vi "play-raster-scan-with-SOS-ID.vi"() -> ()   [LabVIEW 2017]
uses:
  raster-scan-params.ctl
  controls/PI-params.ctl
  controls/boolean_info.ctl
  controls/raster_input_meta_data.ctl
  <vilib>/userdefined/High Color/nirio_resource_hc.ctl
  controls/rasterMetaData.ctl
  <vilib>/Utility/file.llb/Read Delimited Spreadsheet (DBL).vi
  <vilib>/FPGAPlugInAG/cRIO-9082/niLvFpga_Open_cRIO-9082.vi
  <vilib>/rvi/interface/common/dynamic/niFpgaDynamicAddResources.vi
  <vilib>/FPGAPlugInAG/Dynamic/niLvFpga_Reset_Dynamic.vi
  <vilib>/rvi/interface/common/niFpgaWaitOnOcc.vi
  <vilib>/Utility/error.llb/Error Cluster From Error Code.vi
  <vilib>/rvi/errors/niLvFpgaAdjustHostInterfaceError.vi
  <vilib>/FPGAPlugInAG/Dynamic/niLvFpga_Run_Dynamic.vi
  fpga_interface_lib/acquire_FXP_16-5_FIFO_2.vi
  <vilib>/FPGAPlugInAG/Dynamic/niLvFpga_Close_Dynamic.vi
  <userlib>/_matio/level5/Public/Write/Append Data Element.llb/Append Data Element (Anything).vi
  <vilib>/rvi/interface/nirviOpenFPGA/nirviOpenFPGA.xnode
  FPGA Bitfiles/afmimagingcontro_FPGATargetSPARTA_raster-scanning_ejZpyk2O7fU.lvbitx
  <vilib>/rvi/interface/nirviMethod/nirviMethod.xnode
  <vilib>/rvi/interface/nirviReadWriteControl/nirviReadWriteControl.xnode
  <vilib>/rvi/interface/nirviCloseFPGA/nirviCloseFPGA.xnode
  <vilib>/FPGAPlugInAG/Dynamic/niLvFpga_ConfigureFifo_Dynamic.vi
  <vilib>/rvi/errors/niLvFpgaMergeErrorWithErrorCode.vi
  <vilib>/rvi/interface/Simulation/niFpgaSimulationCallBeginRW.vi
  fpga_interface_lib/fpga_interface.lvlib
  NiFpgaLv.dll
  <userlib>/_matio/level5.lvlib
  <vilib>/FPGAPlugInAG/Dynamic/niLvFpga_WriteFifo_Dynamic.vi
panel:
  in  "Ring 2":u16(ring) items=["x(k)", "y(k)", "deflection", "u_z"]
  in  "Alert-on-Finish":bool
  in  "do-Dz":bool
  in  "KI_derate":sgl
  in  "ze_sched_thresh":sgl
  in  "detrend":bool=TRUE
  out "InputMetaData":T1
  out "output-meta-data-path":path
  out "Tab Control":T2(tab)
  in  "Amplitude":dbl=0.15 format="%#_13g"
  in  "Swept-Sines-Control-Settings":cluster{"u-max":sgl, "offset":sgl, "Ki":sgl}
  out "Bode amplitude":cluster{"W":dbl[], "Magnitude":dbl[]}[](graph) caption="Magnitude Graph"
  in  "input-path":path=path "Z:/afm-cs/imaging/raster/5microns/parents/raster_scan_512pix_5mic_01Hz.csv"
  in  "number-of-pixels":i32=512
  out "points_per_line":i32=250000
  out "total_num_points":i32
  in  "raise-constant (init)":sgl
  in  "raise-constant":sgl
  in  "trigger-0":bool
  in  "STOP":bool
  in  "xy-init":fxp<+/-,16,5>[](array[numeric])=[0.0, 0.0]
  in  "Ki-xy":dbl=0.015 format="%#_13g"
  out "ADC-zaxis":sgl
  out "DAC-zaxis":sgl
  in  "xy-bound":sgl=7.0
  out "output-data-path":path
  in  "note-blob":string
  in  "overwrite":bool
  in  "raster-scan-params":T3={"TsTicks"=1600, "Stop"=FALSE, "TOL"=0.3, "ramp-rate"=-0.0002, "z-u-max"=5.0, "PI-params"={"Ki"=0.01, "setpoint"=-0.3}, "Num"=[1.0237086, -2.0434425, 1.0225973, 0.0, 0.0, 0.0, 0.0, 0.0, 0.0], "TF Order"=2, "Den"=[1.0, -1.9961116, 0.998975, 0.0, 0.0, 0.0, 0.0, 0.0, 0.0]} {"ramp-rate" format="%#_5g"; "TOL" format="%#_13g"}
  in  "do_xy_CL":bool=TRUE
  out "boolean errors":T5
  in  "Z-settle-N":i16=10000
  out "Actual Depth":u32
  out "Elements Remaining":u32
  out "size(s)":i32
  out "y iter":i32
  out "nsamps 2":i32
  out "Empty Elements Remaining":u32
  out "(int) y*floor(x/y)":u64
  out "elements left 2":i32=1
  out "x >= y?":bool
  out "writing stopped":bool
  out "size(s) 2":i32
  out "case-selector-feedback":i16
  out "e(0) (threshhold init)":fxp<+/-,16,5>
  out "que timed out?":bool
  out "base y_ref (ramp)":dbl[](graph)
  out "base x_ref(triangle wave)":dbl[](graph)
  out "error":dbl[](graph)
  out "control":dbl[](graph)
  out "x":dbl[](graph)
  out "total-time":dbl
  out "Error signal (previous line) 2":dbl[](graph)
  out "Waveform Graph":dbl[](graph)
  out "Intensity Graph":dbl[][](graph)
  out "control signal (previous line)":dbl[](graph)
  # "x-axis"
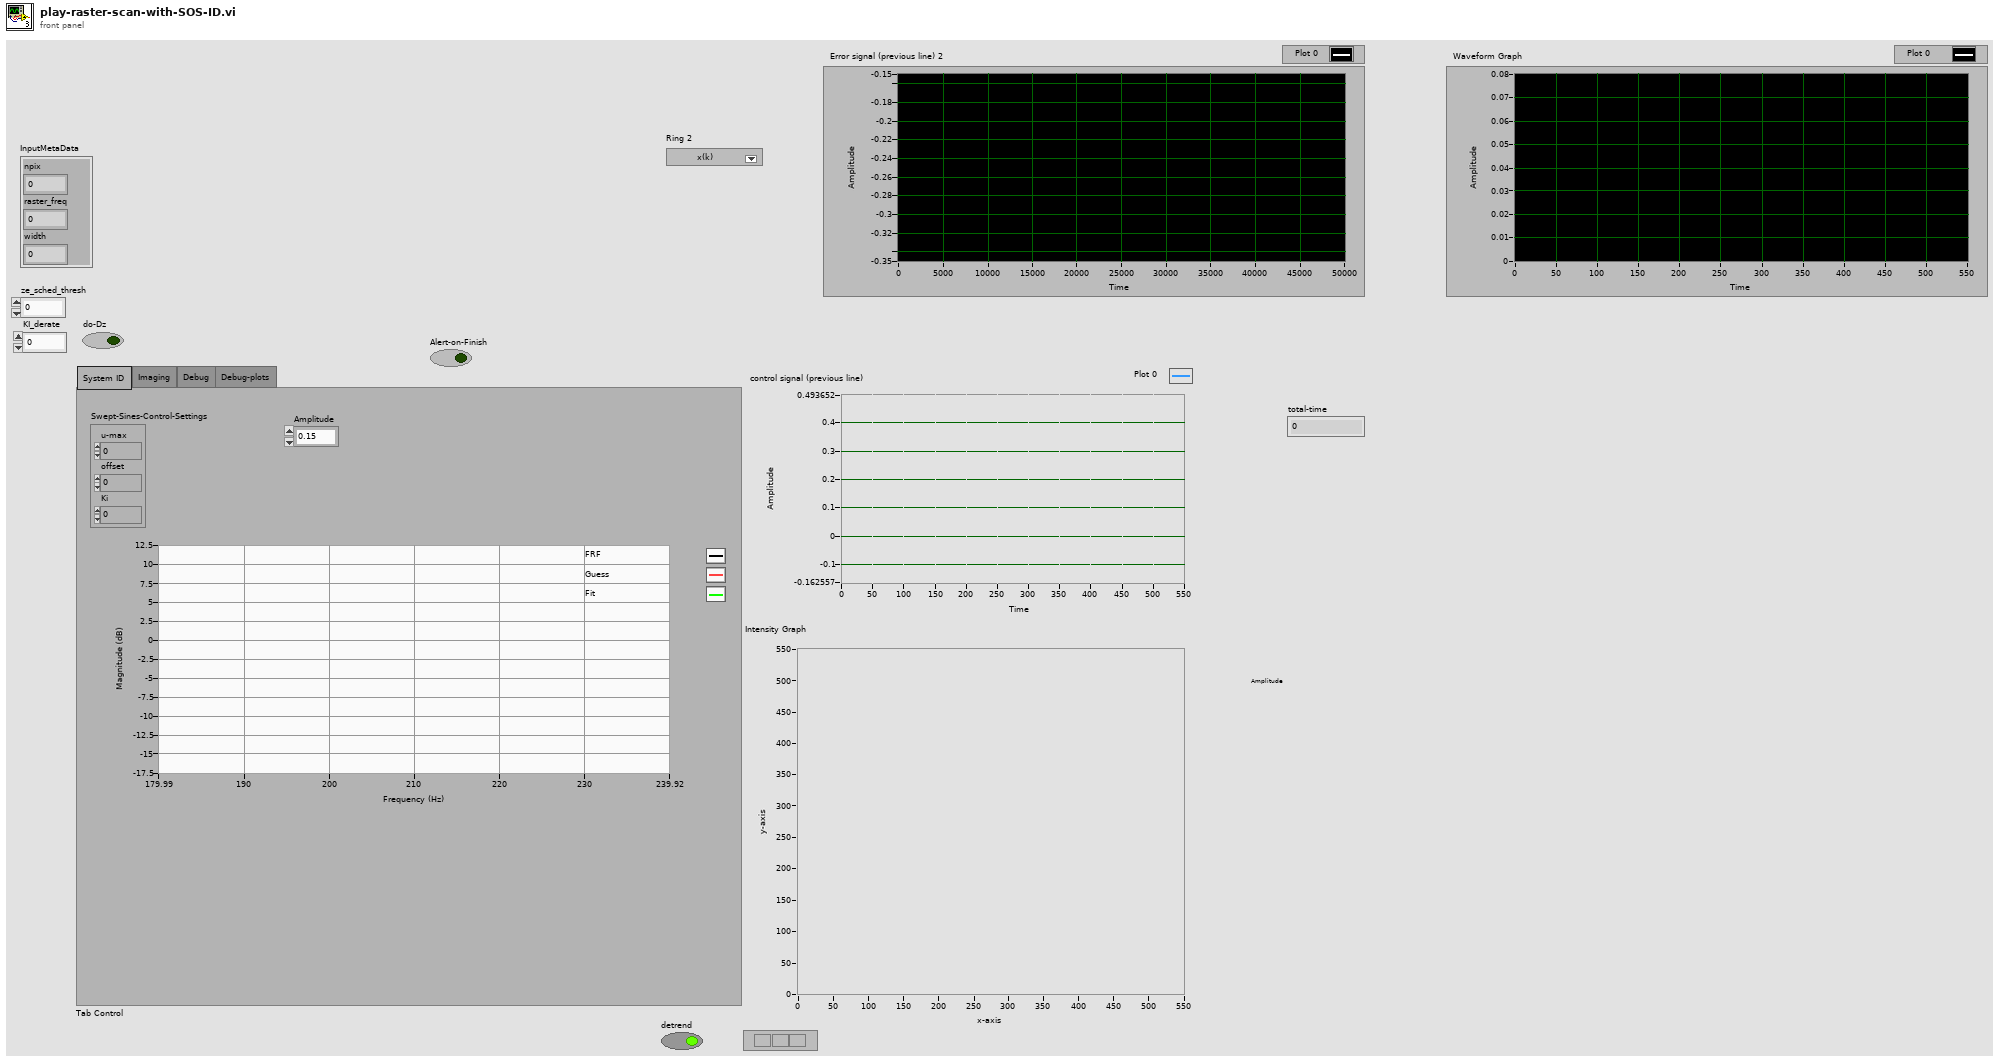
[diagram p1: front panel]
types:
  T1 = typedef "raster_input_meta_data.ctl" = cluster{"npix":dbl, "raster_freq":dbl, "width":dbl}
  T2 = enum32{"System ID", "Imaging", "Debug", "Debug-plots"}
  T3 = typedef "raster-scan-params.ctl" = cluster{"TsTicks":u32, "Stop":bool, "TOL":sgl, "ramp-rate":sgl, "z-u-max":sgl, "PI-params":T4, "Num":sgl[], "TF Order":i32, "Den":sgl[]}
  T4 = typedef "PI-params.ctl" = cluster{"Ki":sgl, "setpoint":sgl}
  T5 = typedef "boolean_info.ctl" = cluster{"unstable-z-traj":bool, "input fifo time-out":bool, "logging fifo timeout":bool, "scanning finished":bool, "unstable-x-traj":bool, "unstable-y-traj":bool, "ABORT":bool, "All Measurements Done":bool, "fpga_finished":bool}
  T6 = typedef "nirio_resource_hc.ctl" = tag
  T7 = typedef "rasterMetaData.ctl" = cluster{"raster-scan-params":T3, "xy-bound":sgl, "DAC-zaxis":sgl, "ADC-zaxis":sgl, "Ki-xy":dbl, "total_num_points":i32, "points_per_line":i32, "number-of-lines":i32, "number-of-pixels":i32, "raster_meta_in":T1, "Ki-derate":sgl, "ze_sched_thresh":sgl}
  T8 = enum16{"open", "replace", "create", "open or create", "replace or create", "replace or create with confirmation"}
  T9 = cluster{"unstable-z-traj":bool, "input fifo time-out":bool, "logging fifo timeout":bool, "scanning finished":bool, "unstable-x-traj":bool, "unstable-y-traj":bool, "ABORT":bool, "All Measurements Done":bool, "fpga_finished":bool}
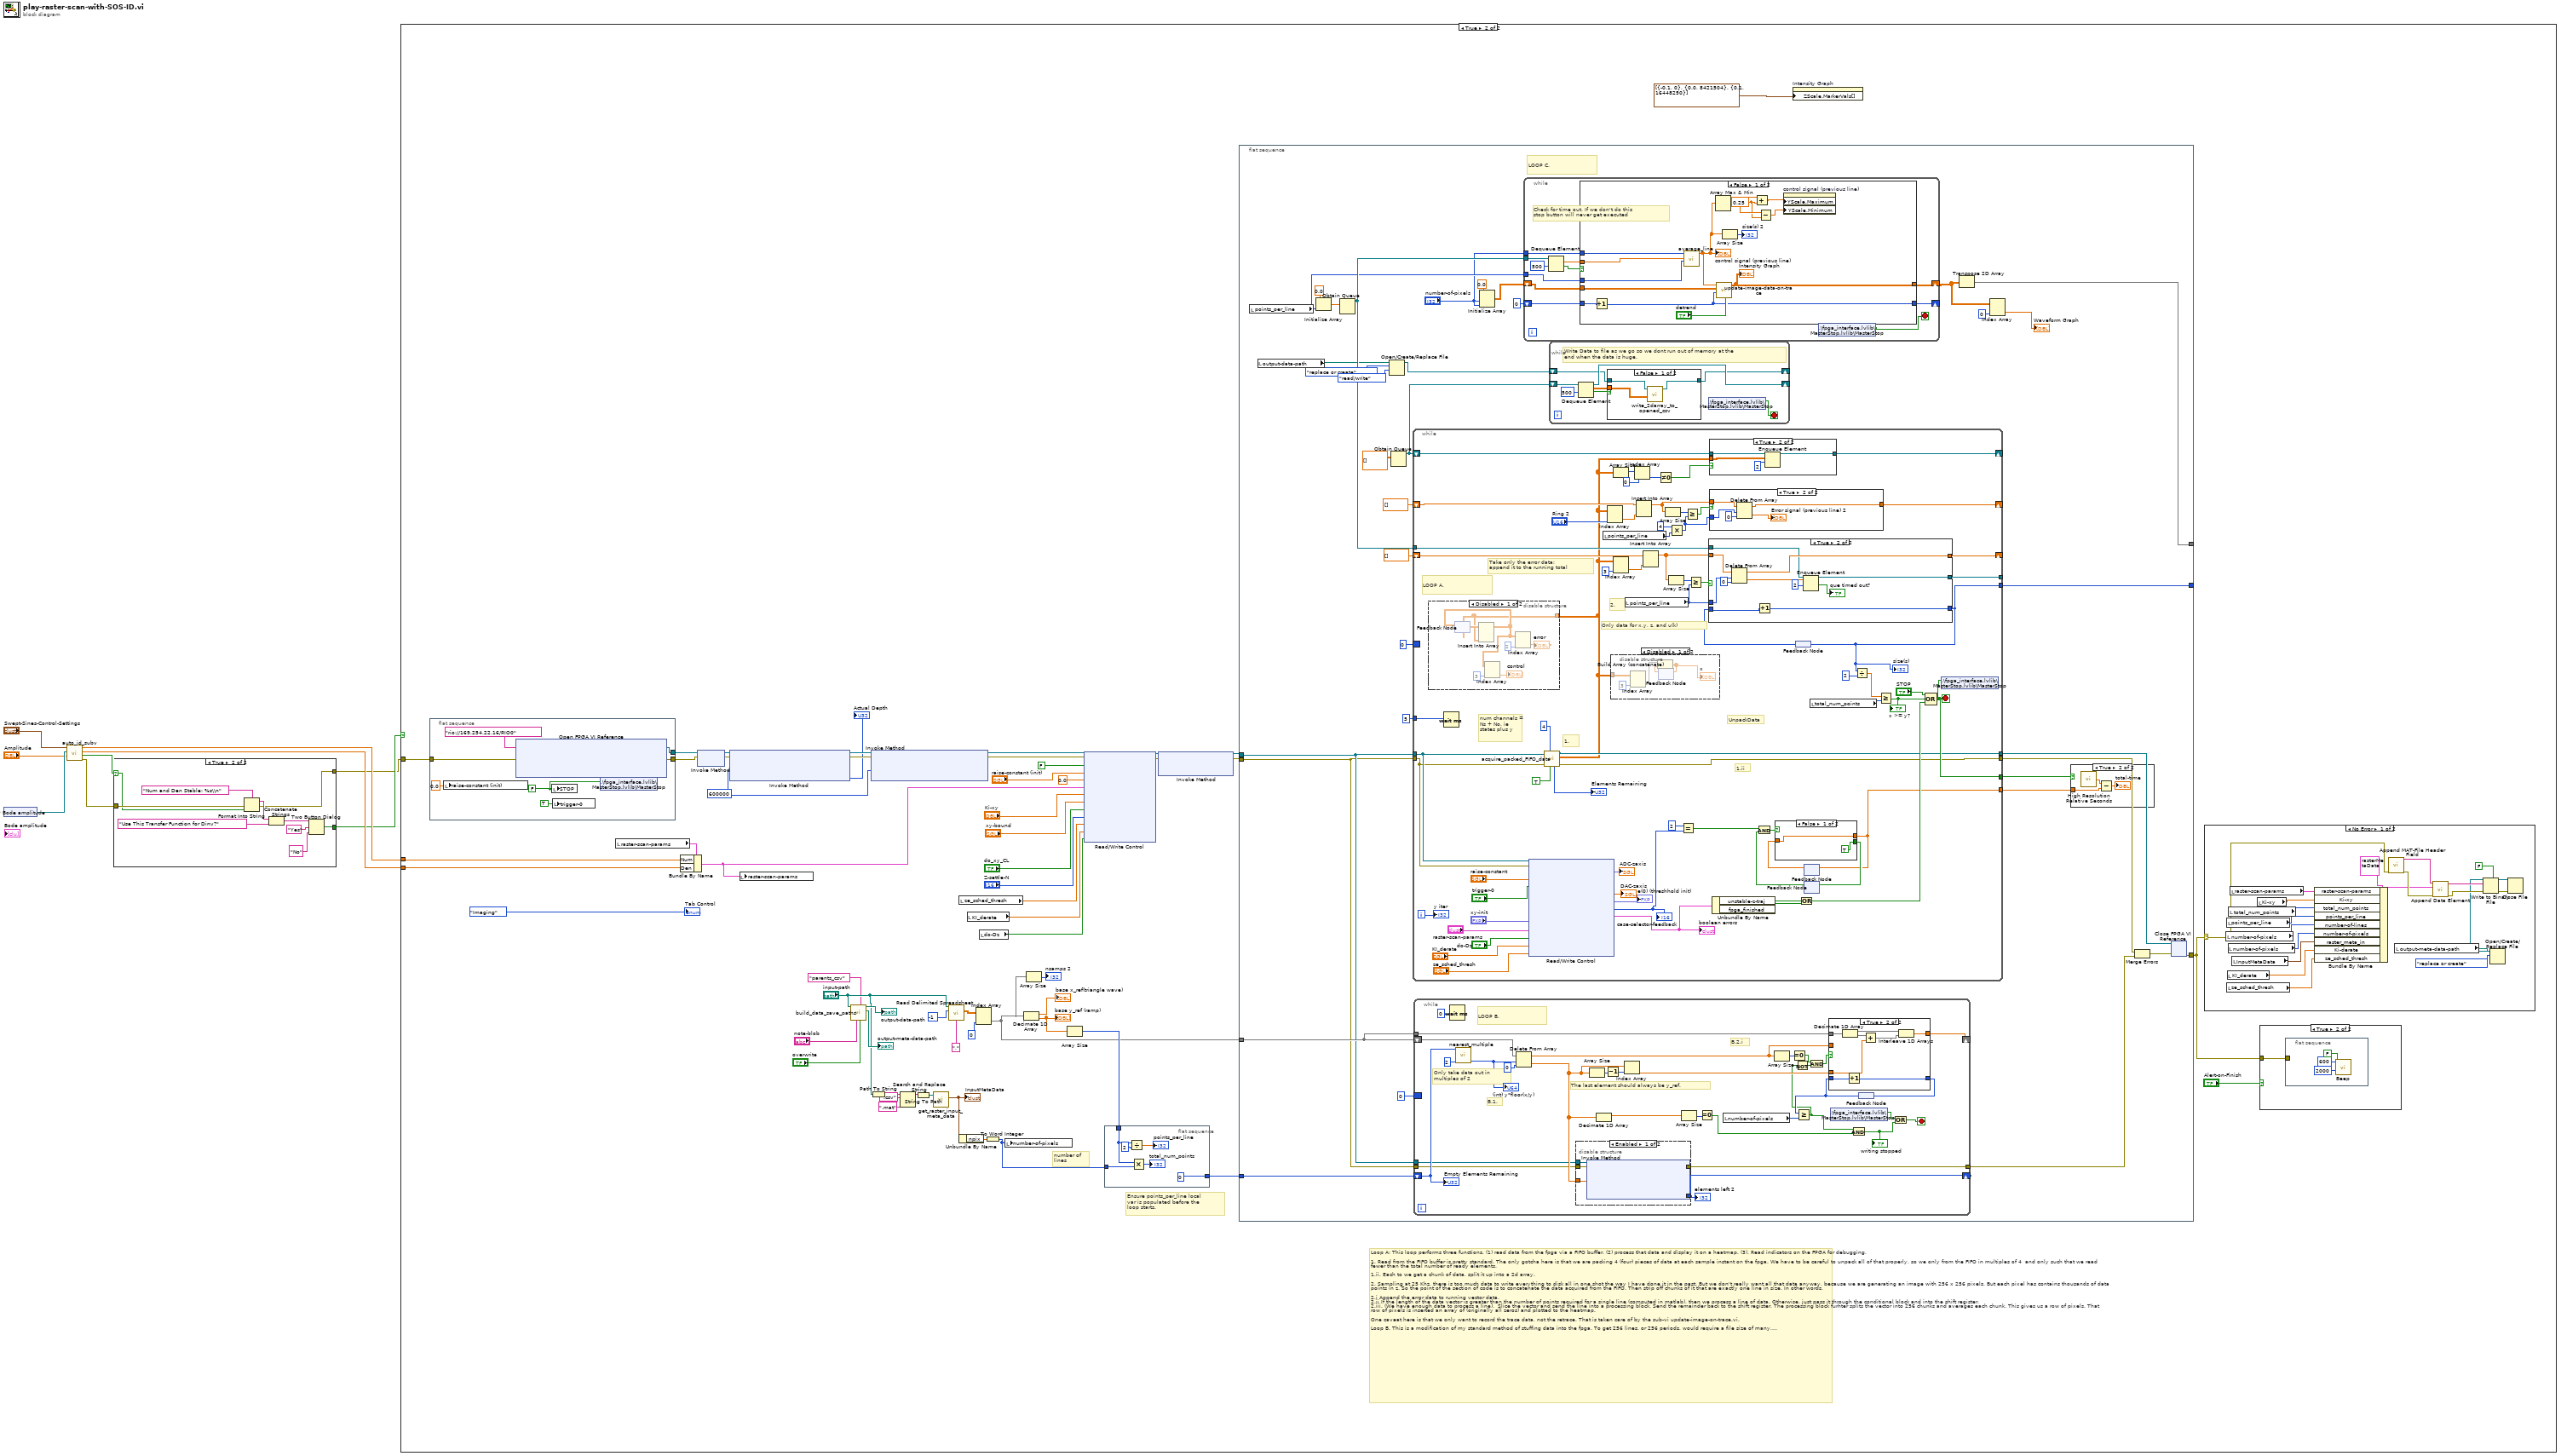
[diagram p0: block diagram]
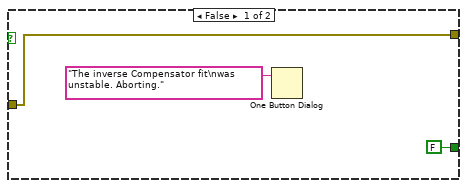
[diagram p2: hidden frame]
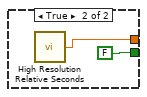
[diagram p13: hidden frame]
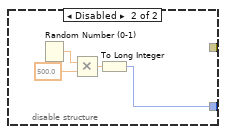
[diagram p16: hidden frame]
diagram:
  n1 = control-ref of="Bode amplitude"() -> (w8:refnum<vi>)
  n2 = call "auto_id_subv.vi"("Amplitude"="Amplitude", "Bode amplitude 2"=w8, "Swept-Sines-Control-Settings"="Swept-Sines-Control-Settings") -> ("error out"=w2:errorcluster, "Is-Totally-Stable"=w1:bool, "Dinv-den"=w5:dbl[], "Dinv-num"=w6:dbl[])  [unwired: 4 in, 1 out]
  n3 = case shown="True" w1 {
    selector: w1 -> [_ w14]
    tunnel: [FALSE ("T button?") w22] -> w4
    tunnel: [w10 w16] -> w3
    tunnel: w2 -> [w10 w15]
    frame False {
      n4 = One Button Dialog(message="The inverse Compensator fit\nwas unstable. Aborting.") -> ()  [unwired: 1 in, 1 out]
    }
    frame True {
      n5 = Format Into String(format string="Num and Den Stable: %s\\n" ("initial string"), error in=w15, w14) -> (resulting string=w18:string, error out=w16:errorcluster)  [unwired: 1 in]
      n6 = Concatenate Strings(w18, "Use This Transfer Function for Dinv?" ("message")) -> (w17:string)
      n7 = Two Button Dialog(message=w17, 1:"No" ("F button name (\"Cancel\")"), 2:"Yes" ("T button name (\"OK\")")) -> (T button?=w22:bool)
    }
  }
  n8 = case shown="True" w4 {
    tunnel: w3 -> [_ w29]
    tunnel: w6 -> [_ w28]
    tunnel: w5 -> [_ w27]
    frame False {
    }
    frame True {
      w77 = 600000
      # "number of \nlines"
      # "Loop A; This loop performs three functions. (1) read data from the fpga via a FIFO buffer. (2) process that data and display it on a heatmap. (3). Read indicators on the FPGA for debugging.\n\n1. Read from the FIFO buffer is pretty standard. The only gotcha here is that we are packing 4 (four) pieces of data at each sample instant on the fpga. We have to be careful to unpack all of that properly, so we only from the FIFO in multiples of 4  and only such that we read fewer than the total number of ready elements. \n\n1.ii. Each to we get a chunk of data, split it up into a 2d array. \n\n2. Sampling at 25 Khz, there is too much data to write everything to disk all in one shot the way I have done it in the past. But we don't really want all that data anyway, because we are generating an image with 256 x 256 pixels. But each pixel has contains thousands of data points in z. So the point of the section of code is to concatenate the data acquired from the FIFO. Then strip off chunks of it that are exactly one line in size. In other words,\n\n2.i Append the error data to running vector data.\n2.ii If the length of the data vector is greater than the number of points required for a single line (computed in matlab), then we process a line of data. Otherwise, just pass it through the conditional block and into the shift register. \n2.iii. (We have enough data to process a line).  Slice the vector and send the line into a processing block. Send the remainder back to the shift register. The processing block furhter splits the vector into 256 chunks and averages each chunk. This gives us a row of pixels. That row of pixels is inserted an array of (originally all zeros) and plotted to the heatmap.\n\nOne caveat here is that we only want to record the trace data, not the retrace. That is taken care of by the sub-vi update-image-on-trace.vi.\n\nLoop B. This is a modification of my standard method of stuffing data into the fpga. To get 256 lines, or 256 periods, would require a file size of many, many gigibtyes. SO the point here is to only use a single period of the triangle wave and corresponding ramp signal. Everytime we exauhst that data, re-cycle the same data and keep pumping it back in. The one tricky part here is that we have to be careful to shift the original ramp data up by the appropriate amount. We also have to take special care because of how the data is packed from matlab. [x(1), y(1), x(2), y(2)...].\n\nThe first iteration of the loop, we don't push any data in. All we do is get the number of empty elements.\n\nB.1 Each iteration, strip off ' empty elements ' elements from the array and send them to FIFO. \nB.2.i Is the remaining array empty?\nB.2.ii Grab the very last element. We need this"
      # "Ensure points_per_line local\nvar is populated before the\nloop starts."
      n9 = flat-sequence {
        tunnel: [w90] -> w76
        tunnel: [w89] -> w75
        tunnel: w29 -> [w86]
        frame #0 {
          w84 = FALSE
          n10 = local write "raise-constant (init)"(0.0) -> ()
          n11 = xnode "Open FPGA VI Reference"("error in"=w86, "resource name"=T6 "rio://169.254.22.16/RIO0") -> ("FPGA VI Reference Out"=w90:refnum<k20>, "error out"=w89:errorcluster)
          n12 = local write "STOP"(w84) -> ()
          n13 = local write "trigger-0"(TRUE ("trigger-0")) -> ()
          n14 = shared-variable ".\\fpga_interface.lvlib\\MasterStop.lvlib\\MasterStop"(w84) -> ()  [unwired: 1 in, 1 out]
        }
      }
      n15 = local read "raster-scan-params"() -> (w26:T3)
      n16 = Bundle By Name(cluster=w26, "Num"=w28, "Den"=w27) -> (w25:T3)
      n17 = xnode "Invoke Method"("FPGA VI Reference In"=w76, "error in"=w75) -> ("FPGA VI Reference Out"=w72:refnum<k20>, "error out"=w71:errorcluster)
      n18 = xnode "Invoke Method"("FPGA VI Reference In"=w72, "error in"=w71, "Requested Depth"=w77) -> ("FPGA VI Reference Out"=w73:refnum<k20>, "error out"=w74:errorcluster, "Actual Depth"=→"Actual Depth":u32)
      n19 = local write "raster-scan-params"(w25) -> ()
      n20 = call "build_data_save_paths.vi"("overwrite"="overwrite", "parent-subfolder-name"="parents_csv", "note-blob"="note-blob", "input-file"="input-path") -> ("output-meta-data-path"=→"output-meta-data-path":path, "output-data-path"=→"output-data-path":path)  [unwired: 4 in, 2 out]
      n21 = Path To String(path="input-path") -> (string=w44:string)
      n22 = xnode "Invoke Method"("FPGA VI Reference In"=w73, "error in"=w74, "Requested Depth"=w77) -> ("FPGA VI Reference Out"=w79:refnum<k20>, "error out"=w78:errorcluster)  [unwired: 1 out]
      n23 = Search and Replace String(input string=w44, search string=".csv", replace string=".mat" ("replace string (\"\")")) -> (result string=w41:string)  [unwired: 5 in, 3 out]
      n24 = String To Path(string=w41) -> (path=w40:path)
      n25 = call "get_raster_input_meta_data.vi"("Path"=w40) -> ("cluster"=w39:T1)  [unwired: 10 in]
      "InputMetaData" <- w39
      n26 = call-poly <vilib>:"Read Delimited Spreadsheet.vi"("file path (dialog if empty)"="input-path", "number of rows (all:-1)"=-1, "delimiter (\\t)"=",") -> ("all rows"=w58:dbl[][])  [unwired: 7 in, 5 out]
      n27 = Unbundle By Name(w39) -> ("npix"=w38:dbl)
      n28 = local read "ze_sched_thresh"() -> (w35:sgl)
      n29 = local read "KI_derate"() -> (w34:sgl)
      n30 = Index Array(array=w58, index (col)=0 ("dimension size")) -> (element=w57:dbl[])  [unwired: 1 in]
      n31 = local read "do-Dz"() -> (w36:bool)
      n32 = To Word Integer(number=w38) -> (16bit integer=w37:i16)
      n33 = local write "number-of-pixels"(w37) -> ()
      n34 = Decimate 1D Array(w57) -> (→"base x_ref(triangle wave)":dbl[], w64:dbl[])
      "base y_ref (ramp)" <- w64
      n35 = Array Size(array=w57) -> (size(s)=→"nsamps 2":i32)
      n36 = Array Size(array=w64) -> (size(s)=w62:i32)
      n37 = xnode "Read/Write Control"("FPGA VI Reference In"=w79, "error in"=w78, "trigger-0"=FALSE ("constant 2 lower"), "raise-constant"="raise-constant (init)", "u(0)"=sgl 0.0, "raster-scan-params"=w25, "Ki-xy"="Ki-xy", "xy-bound"="xy-bound", "do_xy_CL"="do_xy_CL", "Z-settle-N"="Z-settle-N", "ze_sched_thresh"=w35, "KI_derate"=w34, "do-Dz"=w36) -> ("FPGA VI Reference Out"=w54:refnum<k20>, "error out"=w53:errorcluster)
      n38 = flat-sequence {
        tunnel: [0] -> w63
        tunnel: w62 -> [w349]
        tunnel: w37 -> [w352]
        frame #0 {
          n39 = Divide(x=w349, y=2) -> (x/y=→"points_per_line":dbl)
          n40 = Multiply(x=w349, y=w352) -> (x*y=→"total_num_points":i32)
        }
      }
      n41 = xnode "Invoke Method"("FPGA VI Reference In"=w54, "error in"=w53) -> ("FPGA VI Reference Out"=w51:refnum<k20>, "error out"=w52:errorcluster)  [unwired: 1 in]
      n42 = flat-sequence {
        tunnel: [w123] -> _
        tunnel: w51 -> [w132]
        tunnel: w52 -> [w131]
        tunnel: w63 -> [w144]
        tunnel: w57 -> [w133]
        tunnel: [w117] -> _
        tunnel: [w114] -> w31
        frame #0 {
          # "LOOP C."
          n43 = local read "points_per_line"() -> (w129:i32)
          n44 = local read "output-data-path"() -> (w116:path)
          n45 = Initialize Array(0.0 ("element"), w129) -> (w138:dbl[])
          n46 = Obtain Queue(element data type=w138) -> (queue out=w135:refnum<queue>)  [unwired: 4 in, 2 out]
          n47 = Open/Create/Replace File(file path (use dialog)=w116, operation (0:open)=T8."replace or create", access (0:read/write)=enum16{"read/write", "read-only", "write-only"}."read/write") -> (refnum out=w118:refnum<file>)  [unwired: 3 in, 2 out]
          n48 = Obtain Queue(element data type=dbl[][] []) -> (queue out=w121:refnum<queue>)  [unwired: 4 in, 2 out]
          n49 = while {
            tunnel: 5 -> [w256]
            tunnel: w132 -> [w198]
            tunnel: w131 -> [w197]
            tunnel: [w195] -> w126
            tunnel: [w196] -> w127
            shift-right: [w248] -> _
            shift-left: dbl[] [] -> [w246]
            border: 0 ("disabled index (col)") -> [_]
            tunnel: w135 -> [w233]
            tunnel: [w232] -> _
            tunnel: [w199] -> w125
            tunnel: [w201] -> w124
            shift-right: [w219] -> _
            shift-left: w121 -> [w218]
            tunnel: [w217] -> w117
            shift-right: [w205] -> _
            shift-left: dbl[] [] -> [w211]
            i -> [w255]
            stop <- w199 stop-if-true
            # "2."
            # "1.ii"
            # "1."
            # "LOOP A."
            # "Take only the error data;\nappend it to the running total"
            # "num channels = Ns + No, ie states plus y"
            # "Only data for x,y, z, and u(k)"
            # "UnpackData"
            n50 = Wait (ms)(milliseconds to wait=w256) -> ()  [unwired: 1 out]
            n51 = xnode "Read/Write Control"("FPGA VI Reference In"=w198, "error in"=w197, "raise-constant"="raise-constant", "trigger-0"="trigger-0", "xy-init"="xy-init", "raster-scan-params"="raster-scan-params", "do-Dz"="do-Dz", "KI_derate"="KI_derate", "ze_sched_thresh"="ze_sched_thresh") -> ("ADC-zaxis"=→"ADC-zaxis":fxp<+/-,24,5>, "DAC-zaxis"=→"DAC-zaxis":sgl, "e(0) (threshhold init)"=→"e(0) (threshhold init)":fxp<+/-,16,5>, "current-case"=w230:i16, "boolean errors"=w216:T9)  [unwired: 2 out]
            "case-selector-feedback" <- w230
            "boolean errors" <- w216
            n52 = call-poly "acquire_packed_FIFO_data.vi"("Run once?"=TRUE, "numChannels"=u32 4 ("y"), "error in"=w197, "FPGA Interface(in)"=w198) -> ("error out"=w195:errorcluster, "2D Data Out"=w194:dbl[][], "FPGA VI Reference Out"=w196:refnum<k20>, "Elements Remaining"=→"Elements Remaining":u32)  [unwired: 3 in, 1 out]
            n53 = disable-structure shown="Disabled" {
              disable-tunnel: w194 -> [w268 _]
              frame Disabled {
                n54 = feedback #1(w268) -> (w274:dbl[][])
                n55 = Insert Into Array(array=w274, new element=w268) -> (w269:dbl[][])  [unwired: 2 in]
                n56 = feedback-in #1(w269) -> ()
                n57 = Index Array(array=w269, index (col)=3 ("disabled index (col)")) -> (element=→"control":dbl[])  [unwired: 1 in]
                n58 = Index Array(array=w269, index (col)=2 ("disabled index (col)")) -> (element=→"error":dbl[])  [unwired: 1 in]
              }
              frame Enabled {
              }
            }
            n59 = local read "points_per_line"() -> (w209:i32)
            n60 = Index Array(array=w194, index (col)="Ring 2") -> (element=w212:dbl[])  [unwired: 1 in]
            n61 = disable-structure shown="Disabled" {
              disable-tunnel: w194 -> [w266 _]
              frame Disabled {
                n62 = Index Array(array=w266, index (col)=3 ("disabled index (col)")) -> (element=w265:dbl[])  [unwired: 1 in]
                n63 = feedback #2() -> (w264:dbl[])  [unwired: 1 in]
                n64 = Build Array (concatenate)(w265, w264) -> (w263:dbl[])
                "x" <- w263
                n65 = feedback-in #2(w263) -> ()
              }
              frame Enabled {
              }
            }
            n66 = Array Size(array=w194) -> (size(s)=w223:i32[])
            n67 = Index Array(array=w194, index (col)=3 ("disabled index (col)")) -> (element=w245:dbl[])  [unwired: 1 in]
            n68 = local read "points_per_line"() -> (w238:i32)
            n69 = Index Array(array=w223, index=0) -> (element=w221:i32)
            n70 = Insert Into Array(array=w211, new element=w212) -> (w206:dbl[])  [unwired: 1 in]
            n71 = Insert Into Array(array=w246, new element=w245) -> (w224:dbl[])  [unwired: 1 in]
            n72 = Not Equal To 0?(x=w221) -> (x != 0?=w220:bool)
            n73 = Array Size(array=w206) -> (size(s)=w210:i32)
            n74 = Array Size(array=w224) -> (size(s)=w247:i32)
            n75 = Multiply(x=4, y=w209) -> (x*y=w204:i32)
            n76 = Equal?(x=i16 2, y=w230) -> (x = y?=w228:bool)
            n77 = Greater Or Equal?(x=w210, y=w204) -> (x >= y?=w207:bool)
            n78 = Greater Or Equal?(x=w247, y=w238) -> (x >= y?=w244:bool)
            n79 = case shown="True" w220 {
              tunnel: w218 -> [w275 w279]
              tunnel: w194 -> [_ w277]
              tunnel: [w275 w276] -> w219
              frame False {
              }
              frame True {
                n80 = Enqueue Element(queue=w279, element=w277, timeout in ms (-1)=2) -> (queue out=w276:refnum<queue>)  [unwired: 1 in, 2 out]
              }
            }
            n81 = case shown="True" w207 {
              tunnel: w206 -> [w257 w262]
              tunnel: [w257 w259] -> w205
              tunnel: w204 -> [_ w260]
              frame False {
              }
              frame True {
                n82 = Delete From Array(array=w262, length=w260, index=0) -> (deleted portion=→"Error signal (previous line) 2":dbl[], array with subset deleted=w259:dbl[])
              }
            }
            n83 = Unbundle By Name(w216) -> ("unstable-z-traj"=w235:bool, "fpga_finished"=w234:bool)
            n84 = feedback #3() -> (w243:i32)
            n85 = case shown="True" w244 {
              tunnel: [w286 w295] -> w248
              tunnel: w224 -> [w286 w297]
              tunnel: w243 -> [w285 w294]
              tunnel: [w285 w293] -> w217
              tunnel: w238 -> [_ w292]
              tunnel: w233 -> [w284 w290]
              tunnel: [w284 w289] -> w232
              frame False {
              }
              frame True {
                n86 = Delete From Array(array=w297, length=w292, index=0) -> (deleted portion=w291:dbl[], array with subset deleted=w295:dbl[])
                n87 = Increment(x=w294) -> (x+1=w293:i32)
                n88 = Enqueue Element(queue=w290, element=w291, timeout in ms (-1)=2) -> (queue out=w289:refnum<queue>, timed out?=→"que timed out?":bool)  [unwired: 1 in, 1 out]
              }
            }
            "size(s)" <- w217
            n89 = feedback-in #3(w217) -> ()
            n90 = Or(x=w235, y=w234) -> (x .or. y?=w239:bool)
            n91 = feedback #4() -> (w200:dbl)  [unwired: 1 in]
            n92 = feedback #5() -> (w226:bool)  [unwired: 1 in]
            n93 = And(x=w228, y=w226) -> (x .and. y?=w229:bool)
            n94 = case shown="False" w229 {
              tunnel: [TRUE FALSE] -> w227
              tunnel: [w280 w282] -> w201
              tunnel: w200 -> [w280 _]
              frame False {
              }
              frame True {
                n95 = call <vilib>:"High Resolution Relative Seconds.vi"() -> ("relative seconds"=w282:dbl)
              }
            }
            n96 = feedback-in #4(w201) -> ()
            n97 = feedback-in #5(w227) -> ()
            n98 = local read "total_num_points"() -> (w242:i32)
            n99 = Divide(x=w217, y=2) -> (x/y=w237:dbl)
            n100 = Greater Or Equal?(x=w237, y=w242) -> (x >= y?=w240:bool)
            "x >= y?" <- w240
            n101 = Compound Arithmetic op=OR("STOP", w240, w239) -> (w199:bool)
            n102 = shared-variable ".\\fpga_interface.lvlib\\MasterStop.lvlib\\MasterStop"(w199) -> ()  [unwired: 1 in, 1 out]
            "y iter" <- w255
          }
          n103 = while {
            shift-right: [w327] -> _
            shift-left: w144 -> [w323]
            shift-right: [w316] -> _
            shift-left: w133 -> [w328]
            tunnel: w133 -> [w314]
            tunnel: [w320] -> w145
            tunnel: w132 -> [w312]
            tunnel: w131 -> [w311]
            border: 0 ("Timeout (ms)") -> [_]
            stop <- w324 stop-if-true
            # "B.2.i"
            # "B.1."
            # "LOOP B."
            # "Only take data out in \nmultiples of 2"
            # "The last element should always be y_ref."
            n104 = Wait (ms)(milliseconds to wait=0) -> ()  [unwired: 1 out]
            n105 = call "nearest_multiple.vi"("numChan"=u32 2 ("Empty Elements Remaining"), "N"=w323) -> ("(int) y*floor(x/y)"=w322:u64)  [unwired: 9 in]
            "(int) y*floor(x/y)" <- w322
            n106 = Delete From Array(array=w328, length=w322, index=0) -> (deleted portion=w317:dbl[], array with subset deleted=w315:dbl[])
            n107 = disable-structure shown="Enabled" {
              disable-tunnel: [w343 w344] -> w327
              disable-tunnel: w317 -> [w342 _]
              disable-tunnel: [w341 _] -> w320
              disable-tunnel: w312 -> [w340 _]
              disable-tunnel: w311 -> [w339 _]
              frame Enabled {
                n108 = xnode "Invoke Method"("FPGA VI Reference In"=w340, "error in"=w339, "Data"=w342) -> ("error out"=w341:errorcluster, "Empty Elements Remaining"=w343:u32)  [unwired: 1 in, 1 out]
              }
              frame Disabled {
                n109 = Random Number (0-1)() -> (number: 0 to 1=w347:dbl)
                n110 = Multiply(x=w347, y=500.0) -> (x*y=w345:dbl)
                n111 = To Long Integer(number=w345) -> (32bit integer=w344:i32)
              }
            }
            "elements left 2" <- w327
            n112 = Array Size(array=w317) -> (size(s)=w318:i32)
            n113 = Decimate 1D Array(w317) -> (w303:dbl[])  [unwired: 1 out]
            n114 = Decrement(x=w318) -> (x-1=w319:i32)
            n115 = Index Array(array=w317, index=w319) -> (element=w313:dbl)
            n116 = Array Size(array=w303) -> (size(s)=w305:i32)
            n117 = Equal To 0?(x=w305) -> (x = 0?=w304:bool)
            n118 = local read "number-of-pixels"() -> (w309:i32)
            n119 = Array Size(array=w315) -> (size(s)=w325:i32)
            n120 = Equal To 0?(x=w325) -> (x = 0?=w302:bool)
            n121 = shared-variable ".\\fpga_interface.lvlib\\MasterStop.lvlib\\MasterStop"() -> (w298:bool)  [unwired: 1 in, 1 out]
            n122 = feedback #6() -> (w307:i32)
            n123 = Greater Or Equal?(x=w307, y=w309) -> (x >= y?=w300:bool)
            n124 = Not(x=w300) -> (.not. x?=w301:bool)
            n125 = And(x=w302, y=w301) -> (x .and. y?=w299:bool)
            n126 = case shown="True" w299 {
              tunnel: [w330 w333] -> w316
              tunnel: w315 -> [w330 _]
              tunnel: w314 -> [_ w338]
              tunnel: w313 -> [_ w336]
              tunnel: [w329 w332] -> w308
              tunnel: w307 -> [w329 w331]
              frame False {
              }
              frame True {
                n127 = Decimate 1D Array(w338) -> (w335:dbl[], w337:dbl[])
                n128 = Increment(x=w331) -> (x+1=w332:i32)
                n129 = Add(x=w337, y=w336) -> (x+y=w334:dbl[])
                n130 = Interleave 1D Arrays(w335, w334) -> (w333:dbl[])
              }
            }
            n131 = And(x=w300, y=w304) -> (x .and. y?=w306:bool)
            "writing stopped" <- w306
            n132 = feedback-in #6(w308) -> ()
            n133 = Or(x=w298, y=w306) -> (x .or. y?=w324:bool)
            "Empty Elements Remaining" <- w323
          }
          n134 = Initialize Array(0.0 ("element"), "number-of-pixels", "number-of-pixels") -> (w137:dbl[][])
          n135 = while {
            shift-right: [w173] -> w134
            shift-left: w137 -> [w172]
            shift-right: [w170] -> _
            shift-left: 0 ("disabled index (col)") -> [w171]
            tunnel: w129 -> [w169]
            tunnel: w135 -> [w168]
            tunnel: "number-of-pixels" -> [w164]
            stop <- w163 stop-if-true
            # "Check for time out. If we don't do this\nstop button will never get executed"
            n136 = Dequeue Element(queue=w168, timeout in ms (-1)=500) -> (element=w167:dbl[], timed out?=w165:bool)  [unwired: 1 in, 2 out]
            n137 = case shown="False" w165 {
              tunnel: [w188 w189] -> w173
              tunnel: w172 -> [w187 w189]
              tunnel: w171 -> [w186 w190]
              tunnel: [w175 w190] -> w170
              tunnel: w169 -> [w185 _]
              tunnel: w167 -> [w184 _]
              tunnel: w164 -> [w182 _]
              frame False {
                w176 = 0.25
                n138 = Increment(x=w186) -> (x+1=w175:i32)
                n139 = call "average_line.vi"("data-pts-per-line"=w185, "raw-data-row"=w184, "number-of-pixels"=w182) -> ("avg-data-row"=w174:dbl[])  [unwired: 8 in]
                "control signal (previous line)" <- w174
                n140 = Array Max & Min(array=w174) -> (max value=w180:dbl, min value=w177:dbl)  [unwired: 2 out]
                n141 = call "update-image-data-on-trace.vi"("detrend"="detrend", "iterator"=w175, "master-image-data-n"=w187, "avg-data-row"=w174) -> ("master-image-data-out"=w188:dbl[][])  [unwired: 7 in]
                "Intensity Graph" <- w188
                n142 = Array Size(array=w174) -> (size(s)=→"size(s) 2":i32)
                n143 = Add(x=w180, y=w176) -> (x+y=w179:dbl)
                n144 = Subtract(x=w177, y=w176) -> (x-y=w178:dbl)
                n145 = property on="control signal (previous line)" class="WFGraph (strict)"("YScale.Maximum"=w179, "YScale.Minimum"=w178) -> ()  [unwired: 2 in, 2 out]
              }
              frame True {
              }
            }
            n146 = shared-variable ".\\fpga_interface.lvlib\\MasterStop.lvlib\\MasterStop"() -> (w163:bool)  [unwired: 1 in, 1 out]
          }
          n147 = while {
            shift-right: [w151] -> _
            shift-left: w121 -> [w152]
            shift-right: [w149] -> _
            shift-left: w118 -> [w150]
            stop <- w148 stop-if-true
            # "Write Data to file as we go so we dont run out of memory at the \nend when the data is huge."
            n148 = Dequeue Element(queue=w152, timeout in ms (-1)=500) -> (queue out=w151:refnum<queue>, element=w153:dbl[][], timed out?=w154:bool)  [unwired: 1 in, 1 out]
            n149 = case shown="False" w154 {
              tunnel: w153 -> [w156 _]
              tunnel: w150 -> [w158 w159]
              tunnel: [w157 w159] -> w149
              frame False {
                n150 = call "write_2darray_to_opened_csv.vi"("Data_in"=w156, "file_ref_in"=w158) -> ("file_ref_out"=w157:refnum<file>)  [unwired: 8 in, 1 out]
              }
              frame True {
              }
            }
            n151 = shared-variable ".\\fpga_interface.lvlib\\MasterStop.lvlib\\MasterStop"() -> (w148:bool)  [unwired: 1 in, 1 out]
          }
          n152 = Transpose 2D Array(2D array=w134) -> (transposed array=w123:dbl[][])
          n153 = Index Array(array=w134, index (col)=0 ("disabled index (col)")) -> (element=→"Waveform Graph":dbl[])  [unwired: 1 in]
          n154 = case shown="True" w125 {
            tunnel: w124 -> [_ w162]
            frame False {
            }
            frame True {
              n155 = call <vilib>:"High Resolution Relative Seconds.vi"() -> ("relative seconds"=w161:dbl)
              n156 = Subtract(x=w161, y=w162) -> (x-y=→"total-time":dbl)
            }
          }
          n157 = Merge Errors(w126, w145) -> (w115:errorcluster)
          n158 = xnode "Close FPGA VI Reference"("FPGA VI Reference In"=w127, "error in"=w115) -> ("error out"=w114:errorcluster)
        }
      }
      n159 = property on="Intensity Graph" class="IntGraph (strict)"("ZScale.MarkerVals[]"=cluster{dbl, u32}[] [{-0.1, 0}, {0.0, 8421504}, {0.1, 16448250}] ("Z Scale.Marker Values[]")) -> ()  [unwired: 2 in, 2 out]
      n160 = case shown="No Error" w31 {
        selector: w31 -> [w101 _]
        frame No Error {
          n161 = local read "number-of-pixels"() -> (w95:i32)
          n162 = local read "points_per_line"() -> (w96:i32)
          n163 = local read "ze_sched_thresh"() -> (w91:sgl)
          n164 = local read "KI_derate"() -> (w92:sgl)
          n165 = local read "number-of-pixels"() -> (w94:i32)
          n166 = local read "total_num_points"() -> (w97:i32)
          n167 = local read "raster-scan-params"() -> (w99:T3)
          n168 = local read "InputMetaData"() -> (w93:T1)
          n169 = local read "Ki-xy"() -> (w98:dbl)
          n170 = Bundle By Name(cluster=T7 {"raster-scan-params"={"TsTicks"=1600, "Stop"=TRUE, "TOL"=0.3, "ramp-rate"=-5e-05, "z-u-max"=5.0, "PI-params"={"Ki"=0.01, "setpoint"=0.0}, "Num"=[1.0, 0.0, 0.0, 0.0, 0.0, 0.0, 0.0, 0.0, 0.0], "TF Order"=3, "Den"=[1.0, 0.0, 0.0, 0.0, 0.0, 0.0, 0.0, 0.0, 0.0]}, "xy-bound"=7.0, "DAC-zaxis"=0.0, "ADC-zaxis"=0.0, "Ki-xy"=0.01, "total_num_points"=0, "points_per_line"=250000, "number-of-lines"=256, "number-of-pixels"=256, "raster_meta_in"={"npix"=0.0, "raster_freq"=0.0, "width"=0.0}, "Ki-derate"=0.01, "ze_sched_thresh"=0.0} ("Cluster"), "raster-scan-params"=w99, "Ki-xy"=w98, "total_num_points"=w97, "points_per_line"=w96, "number-of-lines"=w95, "number-of-pixels"=w94, "raster_meta_in"=w93, "Ki-derate"=w92, "ze_sched_thresh"=w91) -> (w100:T7)
          n171 = call <userlib>:"Append MAT-File Header Field.vi"("error"=w101) -> ("result string"=w112:string, "error out"=w106:errorcluster)  [unwired: 13 in]
          n172 = local read "output-meta-data-path"() -> (w103:path)
          n173 = call-poly <userlib>:"Append Data Element.vi"("initial string"=w112, "data"=w100, "error in (no error)"=w106) -> ("result string"=w110:string, "error out"=w111:errorcluster)  [unwired: 11 in]
          n174 = Open/Create/Replace File(file path (use dialog)=w103, operation (0:open)=T8."replace or create") -> (refnum out=w105:refnum<file>)  [unwired: 4 in, 2 out]
          n175 = Write to Binary File(file (use dialog)=w105, data=w110, error in=w111, 5:FALSE ("prepend array or string size? (T)")) -> (refnum out=w107:refnum<file>, error out=w108:errorcluster)  [unwired: 2 in, 1 out]
          n176 = Close File(refnum=w107, error in=w108) -> ()  [unwired: 2 out]
        }
        frame Error {
        }
      }
      n177 = case shown="True" "Alert-on-Finish" {
        tunnel: w31 -> [_ w80]
        frame False {
        }
        frame True {
          n178 = flat-sequence {
            tunnel: w80 -> [_]
            frame #0 {
              n179 = call <vilib>:"Beep.vi"("use system alert? (T)"=FALSE, "duration (msec)"=u32 2000, "frequency (Hz)"=u32 600) -> ()  [unwired: 9 in]
            }
          }
        }
      }
      "Tab Control" <- enum32{"System ID", "Imaging", "Debug"}."Imaging" ("Tab Control")
    }
  }
